vi "温度计作业.vi"() -> ()   [LabVIEW 2014]
panel:
  in  "确定按钮":bool
  out "采集进度 3":u8(slide) scale=0.0..10.0
  in  "停止":bool
  out "温度显示器":T1 {"温度计" scale=0.0..100.0}
  in  "温度配置器":cluster{"温度上限(摄氏)":dbl, "摄氏度/华氏度":bool}
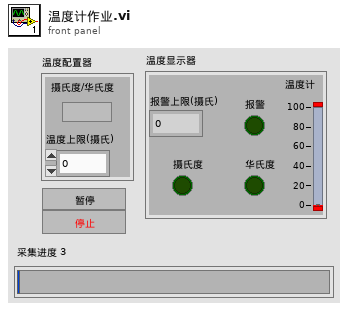
[diagram p1: front panel]
types:
  T1 = cluster{"温度计":dbl, "摄氏度":bool, "报警":bool, "华氏度":bool, "报警上限(摄氏)":dbl}
  T2 = cluster{"温度计":dbl, "摄氏度":bool, "报警":bool, "华氏度":bool, "报警上限":dbl}
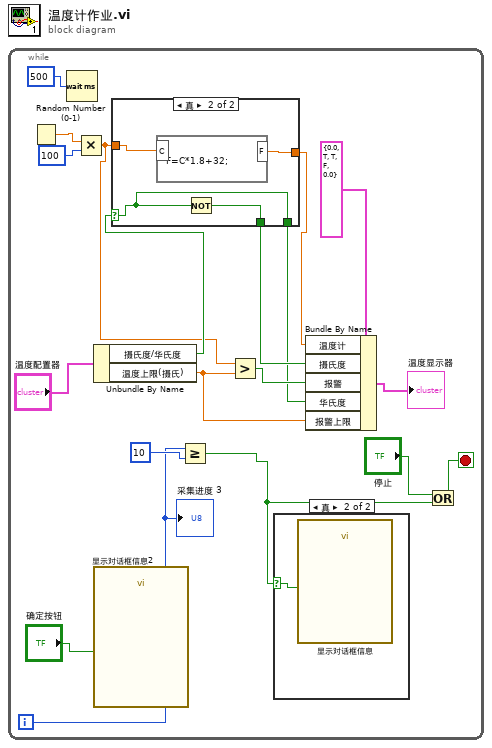
[diagram p0: block diagram]
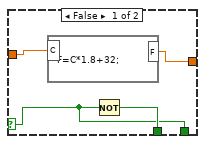
[diagram p3: hidden frame]
diagram:
  n1 = while {
    i -> [w5]
    stop <- w3 stop-if-true
    n2 = Random Number (0-1)() -> (number: 0 to 1=w17:dbl)
    n3 = Wait (ms)(milliseconds to wait=500) -> ()  [unwired: 1 out]
    n4 = Multiply(x=w17, y=100) -> (x*y=w13:dbl)
    n5 = Unbundle By Name("温度配置器") -> ("摄氏度/华氏度"=w15:bool, "温度上限(摄氏)"=w14:dbl)
    n6 = call "显示对话框信息2"("Enable"="确定按钮") -> ()  [unwired: 9 in, 2 out]
    n7 = case shown="真" w15 {
      selector: w15 -> [w21 w27]
      tunnel: w13 -> [w24 w25]
      tunnel: [w22 w28] -> w10
      tunnel: [w21 w27] -> w9
      tunnel: [w23 w26] -> w7
      frame False {
        n8 = formula code="F=C*1.8+32;"("C"=w24) -> ("F"=w23:dbl)
        n9 = Not(x=w21) -> (.not. x?=w22:bool)
      }
      frame True {
        n10 = formula code="F=C*1.8+32;"("C"=w25) -> ("F"=w26:dbl)
        n11 = Not(x=w27) -> (.not. x?=w28:bool)
      }
    }
    n12 = Greater Or Equal?(x=w5, y=10) -> (x >= y?=w1:bool)
    n13 = Greater?(x=w13, y=w14) -> (0:w12:bool)
    n14 = case shown="真" w1 {
      selector: w1 -> [_ w20]
      frame False {
      }
      frame True {
        n15 = call "显示对话框信息"("Enable"=w20) -> ()  [unwired: 9 in, 2 out]
      }
    }
    n16 = Bundle By Name(cluster=T2 {"温度计"=0.0, "摄氏度"=TRUE, "报警"=TRUE, "华氏度"=FALSE, "报警上限"=0.0}, "温度计"=w7, "摄氏度"=w10, "报警"=w12, "华氏度"=w9, "报警上限"=w14) -> (→"温度显示器":T2)
    n17 = Or(x="停止", y=w1) -> (x .or. y?=w3:bool)
    "采集进度 3" <- w5
  }
